vi "NUSP2val.vi"(8 "error in":errorcluster, 10 "Número USP":dbl=4112767.0 format="%#_13g", 11 "Exercise Number":u32) -> (0 "error out":errorcluster, 3 "Waveform Out":waveform(dbl))   [LabVIEW 2014]
uses:
  Ctls/ExerciseWfmType.ctl
  <vilib>/Analysis/4window.llb/Exponential Window (DBL).vi
  <vilib>/measure/NI_MABase.lvlib
  <vilib>/measure/NI_MAPro.lvlib
  <vilib>/Analysis/NI_AALBase.lvlib
  <vilib>/Analysis/NI_AALPro.lvlib
panel:
  out "Waveform Graph":waveform(dbl)(graph)
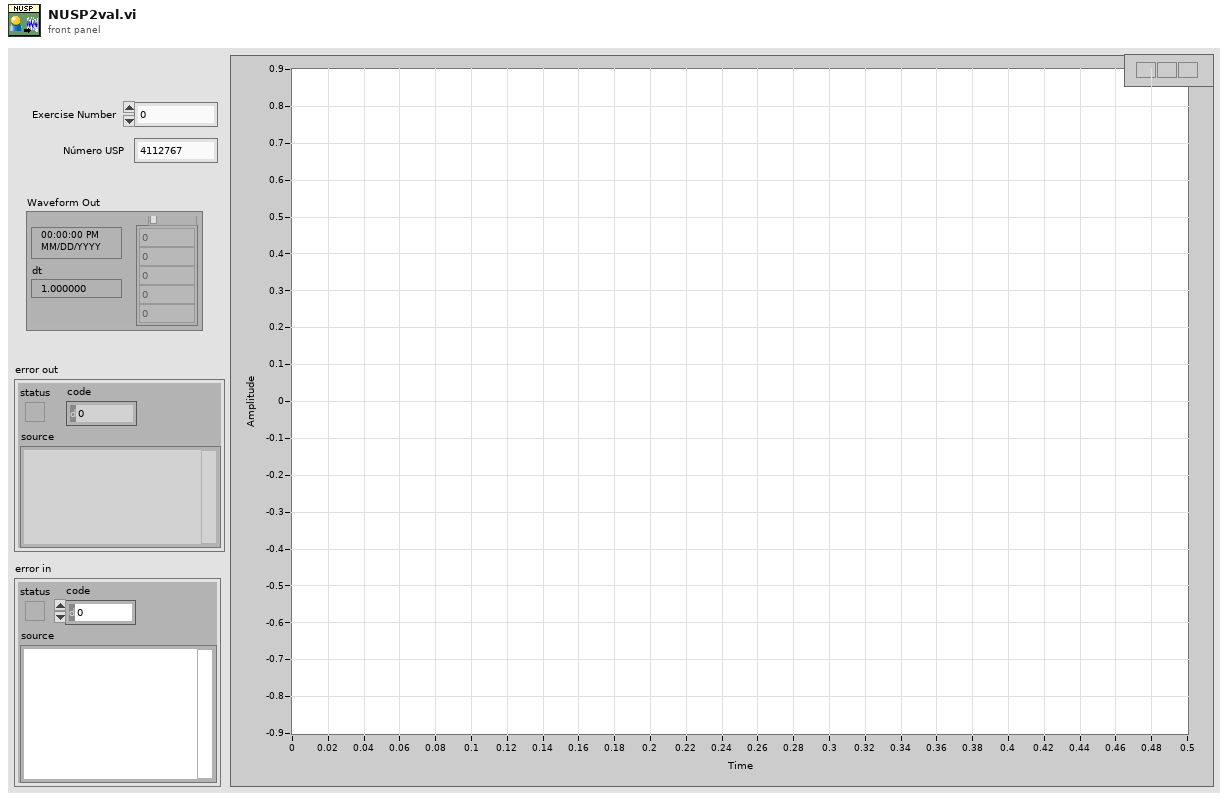
[diagram p1: front panel]
types:
  T1 = cluster{"standard deviation":dbl, "F1delta":dbl, "F2delta":dbl, "F3delta":dbl, "A1delta":dbl, "A2delta":dbl, "A3delta":dbl, "A3min":dbl, "A2min":dbl, "A1min":dbl, "F3min":dbl, "F2min":dbl, "F1min":dbl}
  T2 = typedef "ExerciseWfmType.ctl" = enum16{"Multitone", "Chirp", "Square Wave"}
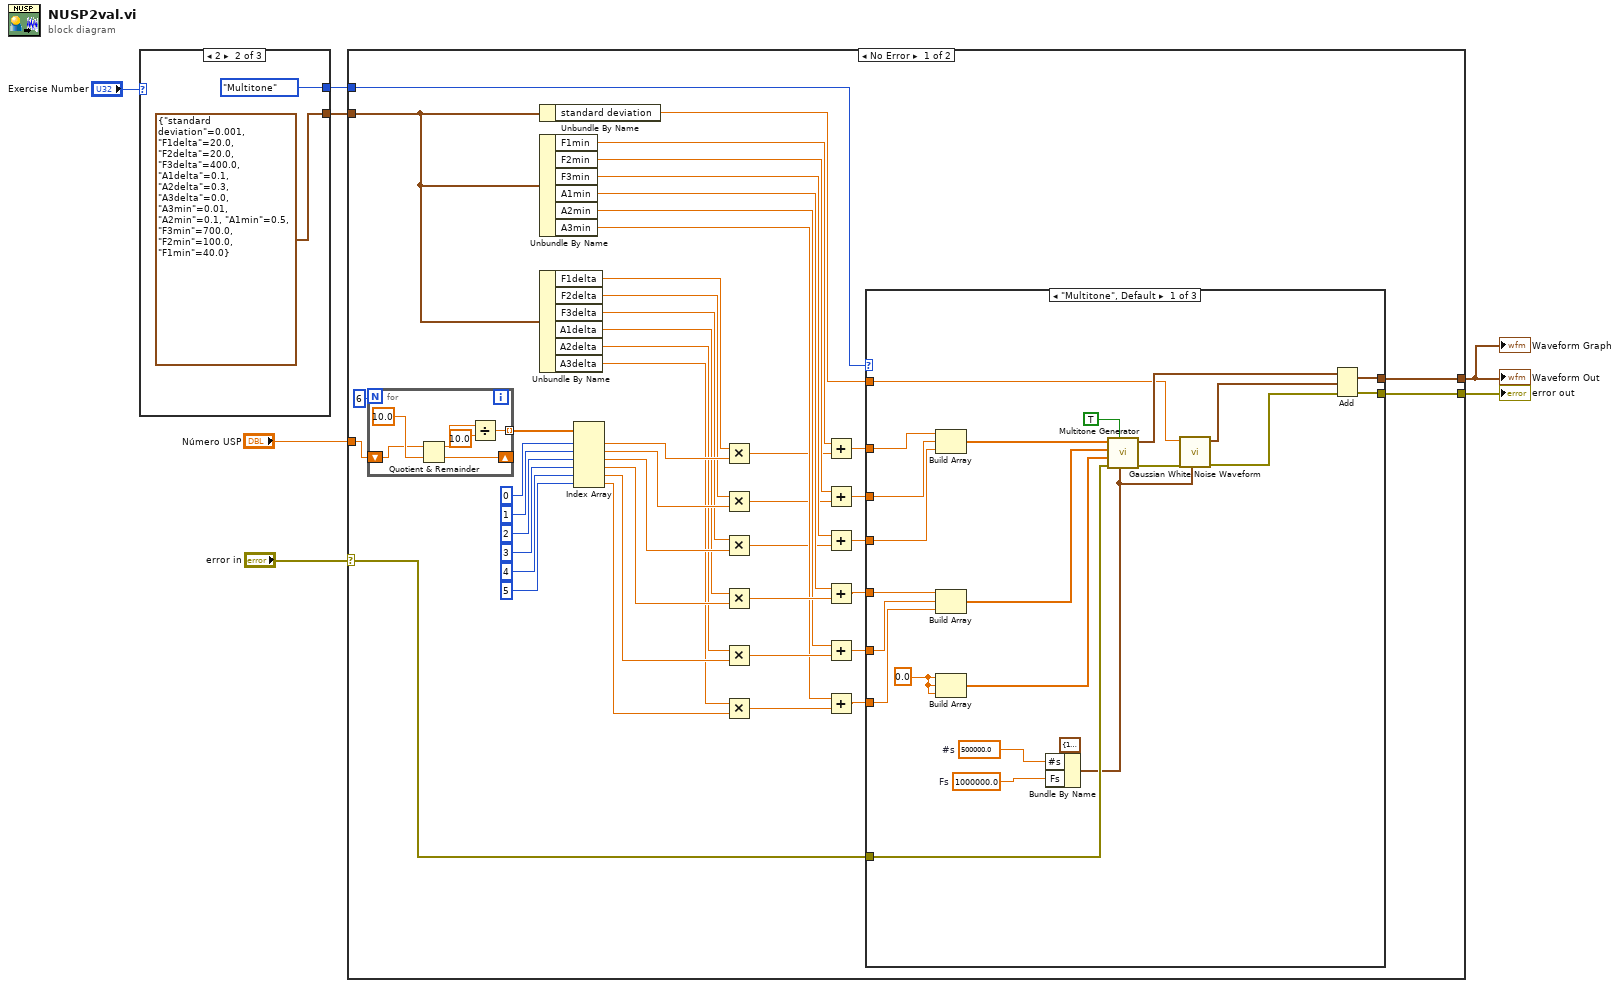
[diagram p0: block diagram]
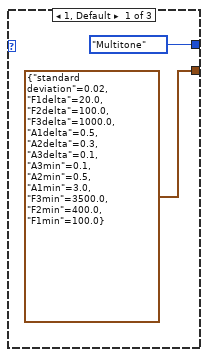
[diagram p2: hidden frame]
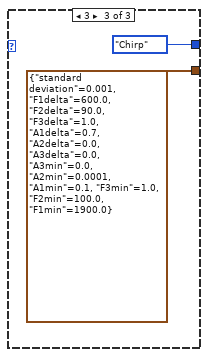
[diagram p3: hidden frame]
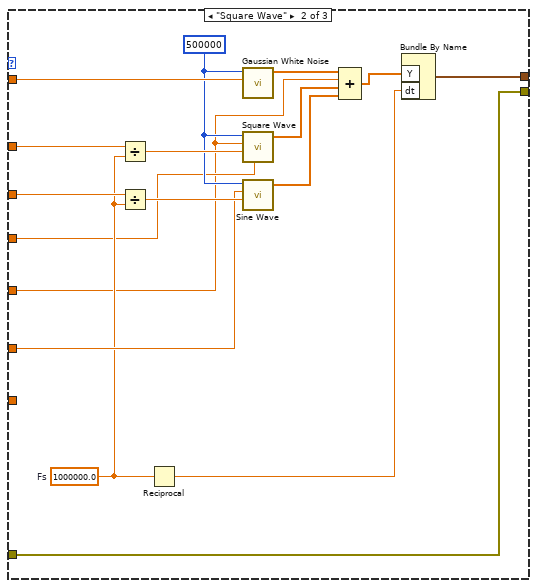
[diagram p4: hidden frame]
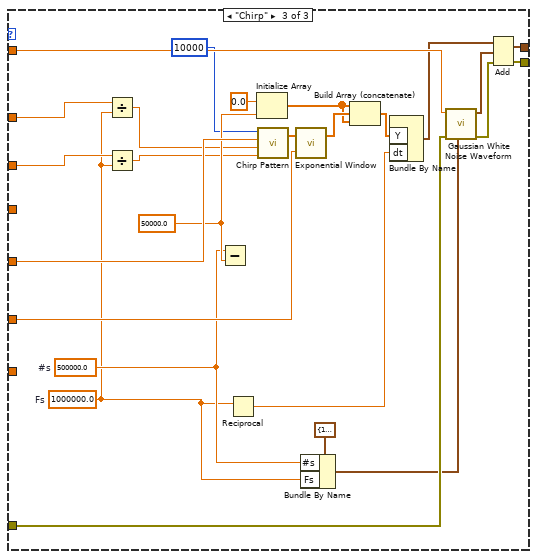
[diagram p5: hidden frame]
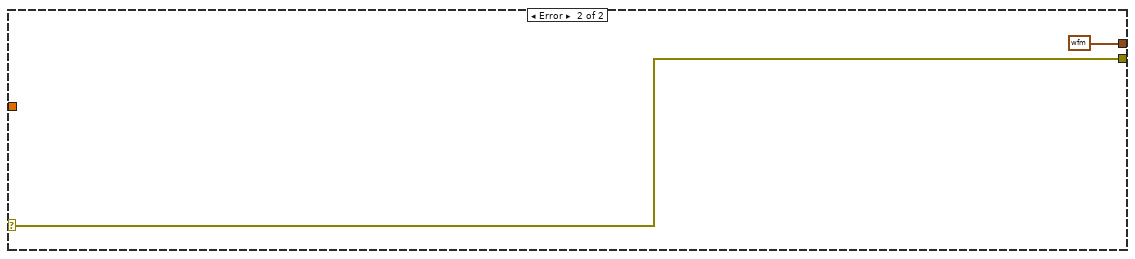
[diagram p6: hidden frame]
diagram:
  n1 = case shown="2" "Exercise Number" {
    tunnel: [T1 {"standard deviation"=0.02, "F1delta"=20.0, "F2delta"=100.0, "F3delta"=1000.0, "A1delta"=0.5, "A2delta"=0.3, "A3delta"=0.1, "A3min"=0.1, "A2min"=0.5, "A1min"=3.0, "F3min"=3500.0, "F2min"=400.0, "F1min"=100.0} ("F & A") T1 {"standard deviation"=0.001, "F1delta"=20.0, "F2delta"=20.0, "F3delta"=400.0, "A1delta"=0.1, "A2delta"=0.3, "A3delta"=0.0, "A3min"=0.01, "A2min"=0.1, "A1min"=0.5, "F3min"=700.0, "F2min"=100.0, "F1min"=40.0} ("F & A") T1 {"standard deviation"=0.001, "F1delta"=600.0, "F2delta"=90.0, "F3delta"=1.0, "A1delta"=0.7, "A2delta"=0.0, "A3delta"=0.0, "A3min"=0.0, "A2min"=0.0001, "A1min"=0.1, "F3min"=1.0, "F2min"=100.0, "F1min"=1900.0} ("F & A")] -> w3
    tunnel: [ExerciseWfmType."Multitone" ExerciseWfmType."Multitone" ExerciseWfmType."Chirp"] -> w2
    frame 1, Default {
    }
    frame 2 {
    }
    frame 3 {
    }
  }
  n2 = case shown="No Error" "error in" {
    selector: "error in" -> [w14 w131]
    tunnel: "Número USP" -> [w55 _]
    tunnel: [w39 w131] -> w5
    tunnel: [w40 waveform(dbl) {"t0"=timestamp(0 s since 1904-01-01), "dt"=1.0, "Y"=[]}] -> w4
    tunnel: w3 -> [w32 _]
    tunnel: w2 -> [w15 _]
    frame No Error {
      n3 = for {
        N: 6 -> [_]
        tunnel: [w124] -> w53 mode=indexing
        shift-right: [w127] -> _
        shift-left: w55 -> [w128]
        n4 = Quotient & Remainder(x=w128, y=10.0) -> (x-y*floor(x/y)=w126:dbl, floor(x/y)=w127:dbl)
        n5 = Divide(x=w126, y=10.0) -> (x/y=w124:dbl)
      }
      n6 = Unbundle By Name(w32) -> ("standard deviation"=w19:dbl)
      n7 = Unbundle By Name(w32) -> ("F1min"=w25:dbl, "F2min"=w24:dbl, "F3min"=w23:dbl, "A1min"=w22:dbl, "A2min"=w21:dbl, "A3min"=w20:dbl)
      n8 = Unbundle By Name(w32) -> ("F1delta"=w31:dbl, "F2delta"=w30:dbl, "F3delta"=w29:dbl, "A1delta"=w28:dbl, "A2delta"=w27:dbl, "A3delta"=w26:dbl)
      n9 = Index Array(array=w53, index #1=0 ("index"), index #2=1 ("index"), index #3=2 ("index"), index #4=3 ("index"), index #5=4 ("index"), index #6=5 ("index")) -> (element #1=w52:dbl, element #2=w51:dbl, element #3=w50:dbl, element #4=w49:dbl, element #5=w48:dbl, element #6=w47:dbl)
      n10 = Multiply(x=w31, y=w52) -> (x*y=w16:dbl)
      n11 = Multiply(x=w30, y=w51) -> (x*y=w17:dbl)
      n12 = Multiply(x=w29, y=w50) -> (x*y=w18:dbl)
      n13 = Multiply(x=w28, y=w49) -> (x*y=w58:dbl)
      n14 = Multiply(x=w27, y=w48) -> (x*y=w57:dbl)
      n15 = Multiply(x=w26, y=w47) -> (x*y=w56:dbl)
      n16 = Add(x=w25, y=w16) -> (x+y=w35:dbl)
      n17 = Add(x=w24, y=w17) -> (x+y=w34:dbl)
      n18 = Add(x=w23, y=w18) -> (x+y=w33:dbl)
      n19 = Add(x=w22, y=w58) -> (x+y=w36:dbl)
      n20 = Add(x=w21, y=w57) -> (x+y=w37:dbl)
      n21 = Add(x=w20, y=w56) -> (x+y=w38:dbl)
      n22 = case shown="\"Multitone\", Default" w15 {
        tunnel: [w73 w87 w121] -> w40
        tunnel: [w71 w86 w120] -> w39
        tunnel: w38 -> [w70 _ _]
        tunnel: w37 -> [w69 w94 w118]
        tunnel: w36 -> [w68 w82 w119]
        tunnel: w35 -> [w65 w98 w103]
        tunnel: w34 -> [w64 w97 w102]
        tunnel: w33 -> [w63 w85 _]
        tunnel: w19 -> [w67 w93 w117]
        tunnel: w14 -> [w66 w86 w114]
        frame "Multitone", Default {
          w60 = 500000.0  # #s
          w61 = 1000000.0  # Fs
          w76 = 0.0 ("element")
          n23 = Build Array(w65, w64, w63) -> (w79:dbl[])
          n24 = Build Array(w68, w69, w70) -> (w81:dbl[])
          n25 = Build Array(w76, w76, w76) -> (w80:dbl[])
          n26 = Bundle By Name(cluster=cluster{"Fs":dbl, "#s":dbl} {"Fs"=1000.0, "#s"=1000.0} ("sampling info"), "#s"=w60, "Fs"=w61) -> (w59:cluster{"Fs":dbl, "#s":dbl})
          n27 = call <vilib>:"Multitone Generator.vi"("sampling info"=w59, "reset signal"=TRUE, "error in (no error)"=w66, "tone phases"=w80, "tone amplitudes"=w81, "tone frequencies"=w79) -> ("error out"=w77:errorcluster, "signal out"=w74:waveform(dbl))  [unwired: 2 in, 2 out]
          n28 = call <vilib>:"Gaussian White Noise Waveform.vi"("sampling info"=w59, "error in (no error)"=w77, "standard deviation"=w67) -> ("error out"=w72:errorcluster, "signal out"=w75:waveform(dbl))  [unwired: 7 in]
          n29 = Add(1:w75, 2:w74, 4:w72) -> (0:w73:waveform(dbl), 3:w71:errorcluster)
        }
        frame "Square Wave" {
          w92 = 500000 ("samples")
          w90 = 1000000.0  # Fs
          n30 = Divide(x=w98, y=w90) -> (x/y=w96:dbl)
          n31 = Divide(x=w97, y=w90) -> (x/y=w95:dbl)
          n32 = Reciprocal(x=w90) -> (1/x=w89:dbl)
          n33 = call <vilib>:"Gaussian White Noise.vi"("standard deviation"=w93, "samples"=w92) -> ("Gaussian noise pattern"=w91:dbl[])  [unwired: 8 in, 1 out]
          n34 = call <vilib>:"Square Wave.vi"("samples"=w92, "amplitude"=w82, "frequency"=w96, "duty cycle (%)"=w85) -> ("square wave"=w84:dbl[])  [unwired: 2 in, 2 out]
          n35 = call <vilib>:"Sine Wave.vi"("samples"=w92, "amplitude"=w94, "frequency"=w95) -> ("sine wave"=w83:dbl[])  [unwired: 2 in, 2 out]
          n36 = Compound Arithmetic op=ADD(w91, w82, w84, w83) -> (w88:dbl[])
          n37 = Bundle By Name("Y"=w88, "dt"=w89) -> (w87:waveform(dbl))  [unwired: 1 in]
        }
        frame "Chirp" {
          w104 = 500000.0  # #s
          w101 = 1000000.0  # Fs
          w112 = 50000.0 ("y")
          n38 = Divide(x=w103, y=w101) -> (x/y=w100:dbl)
          n39 = Divide(x=w102, y=w101) -> (x/y=w99:dbl)
          n40 = Subtract(x=w104, y=w112) -> ()  [unwired: 1 out]
          n41 = Reciprocal(x=w101) -> (1/x=w116:dbl)
          n42 = Initialize Array(0.0 ("element"), w112) -> (w106:dbl[])
          n43 = call <vilib>:"Chirp Pattern.vi"("f2"=w99, "f1"=w100, "amplitude"=w119, "samples"=10000) -> ("Chirp Pattern"=w109:dbl[])  [unwired: 1 out]
          n44 = call-poly <vilib>:"Exponential Window.vi"("final value"=w118, "X"=w109) -> ("Windowed X"=w108:dbl[])  [unwired: 1 out]
          n45 = Bundle By Name(cluster=cluster{"Fs":dbl, "#s":dbl} {"Fs"=1000.0, "#s"=1000.0} ("sampling info"), "#s"=w104, "Fs"=w101) -> (w113:cluster{"Fs":dbl, "#s":dbl})
          n46 = Build Array (concatenate)(w106, w108, w106) -> (w107:dbl[])
          n47 = Bundle By Name("Y"=w107, "dt"=w116) -> (w115:waveform(dbl))  [unwired: 1 in]
          n48 = call <vilib>:"Gaussian White Noise Waveform.vi"("sampling info"=w113, "error in (no error)"=w114, "standard deviation"=w117) -> ("error out"=w122:errorcluster, "signal out"=w123:waveform(dbl))  [unwired: 7 in]
          n49 = Add(1:w123, 2:w115, 4:w122) -> (0:w121:waveform(dbl), 3:w120:errorcluster)
        }
      }
    }
    frame Error {
    }
  }
  "error out" <- w5
  "Waveform Out" <- w4
  "Waveform Graph" <- w4
